vi "FitLorentzien.vi"() -> ()   [LabVIEW 2019]
uses:
  <vilib>/gmath/NumericalOptimization/Nonlinear Curve Fit LM formula string.vi
  <vilib>/Analysis/NI_AALBase.lvlib
  <vilib>/gmath/NI_Gmath.lvlib
panel:
  out "Residuals2":dbl
  out "NLCoeff2":dbl[](array[numeric])
  out "XY Graph 2":cluster{dbl[], "best nonlinear fit":dbl[]}[](graph)
  in  "Stop":bool
  out "Slide":u8(slide) scale=0.0..100.0
  out "Histogram Graph":T1(graph)
  in  "c":dbl
  out "XY Graph":cluster{dbl[], "Array":dbl[]}[](graph)
  out "NLCoeff":dbl[](array[numeric])
  out "Residuals":dbl[](array[numeric])
  out "Best Fit":dbl[](array[numeric])
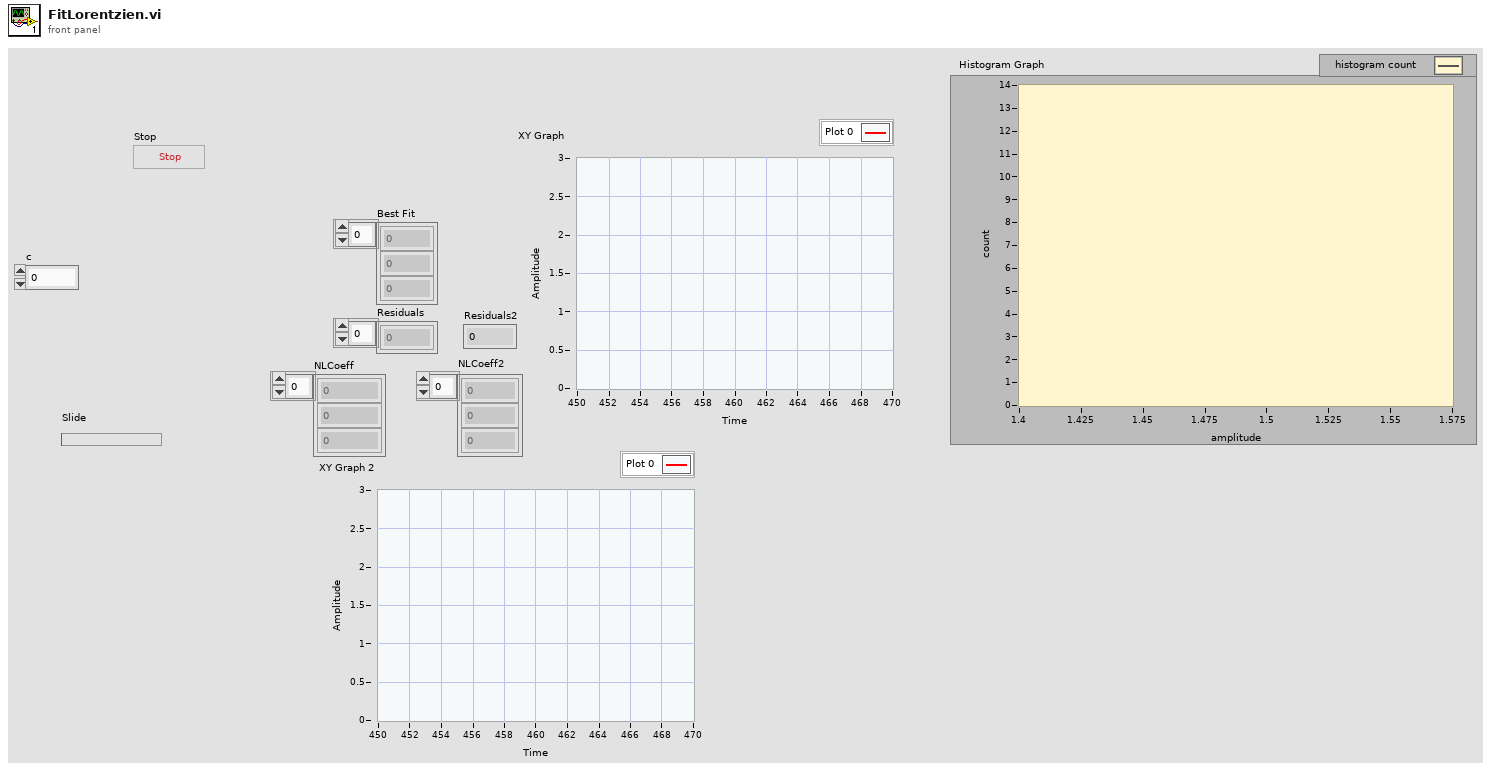
[diagram p1: front panel]
types:
  T1 = cluster{"X Values":dbl[], "Histogram: h(x)":i32[]}
  T2 = cluster{"model":string, "Parameters":string[], "x":string}
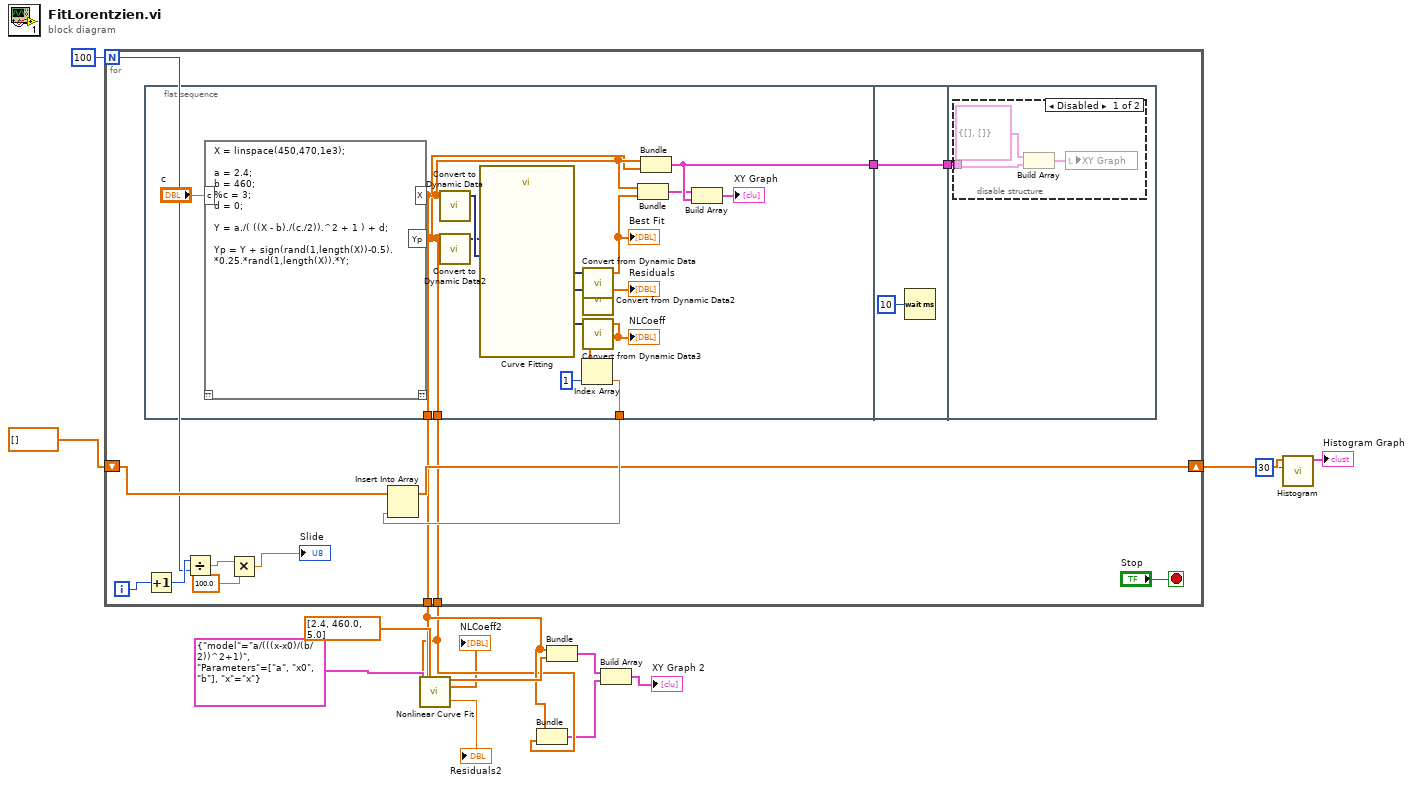
[diagram p0: block diagram]
diagram:
  n1 = for {
    N: 100 -> [w24]
    shift-right: [w27] -> w14
    shift-left: dbl[] [] -> [w29]
    tunnel: [w17] -> w6
    tunnel: [w16] -> w5
    i -> [w26]
    stop <- "Stop" stop-if-true
    n2 = flat-sequence {
      tunnel: [w45] -> w19
      tunnel: [w32] -> w28
      tunnel: [w31] -> w17
      tunnel: [w30] -> w16
      tunnel: w19 -> [w47]
      tunnel: [w47] -> w18
      tunnel: w18 -> [w48]
      frame #0 {
        n3 = script code="X = linspace(450,470,1e3);\n\na = 2.4;\nb = 460;\n%c = 3;\nd = 0;\n\nY = a./( ((X - b)./(c./2)).^2 + 1 ) + d;\n\nYp = Y + sign(rand(1,length(X))-0.5).*0.25.*rand(1,length(X)).*Y;"("c"="c") -> ("Yp"=w30:dbl[], "X"=w31:dbl[])  [unwired: 1 in, 1 out]
        n4 = call "Convert to Dynamic Data"("Array"=w31) -> ("Dynamic Data Type"=w44:dynamicdata)  [unwired: 3 in]
        n5 = call "Convert to Dynamic Data2"("Array"=w30) -> ("Dynamic Data Type"=w43:dynamicdata)  [unwired: 3 in]
        n6 = call "Curve Fitting"("Locations"=w44, "Signals"=w43) -> ("residual"=w41:dynamicdata, "best fit"=w42:dynamicdata, "non-linear coefficients"=w39:dynamicdata)  [unwired: 5 in, 2 out]
        n7 = call "Convert from Dynamic Data"("Dynamic Data Type"=w42) -> ("Array"=w38:dbl[])  [unwired: 3 in]
        "Best Fit" <- w38
        n8 = call "Convert from Dynamic Data2"("Dynamic Data Type"=w41) -> ("Array"=→"Residuals":dbl[])  [unwired: 3 in]
        n9 = call "Convert from Dynamic Data3"("Dynamic Data Type"=w39) -> ("Array"=w34:dbl[])  [unwired: 3 in]
        "NLCoeff" <- w34
        n10 = Index Array(array=w34, index=1) -> (element=w32:dbl)
        n11 = Bundle(w31, "Array"=w38) -> (w35:cluster{dbl[], "Array":dbl[]})  [unwired: 1 in]
        n12 = Bundle(w31, w30) -> (w45:cluster{dbl[], dbl[]})  [unwired: 1 in]
        n13 = Build Array(w35, w45) -> (→"XY Graph":cluster{dbl[], "Array":dbl[]}[])
      }
      frame #1 {
        n14 = Wait (ms)(milliseconds to wait=u32 10) -> ()  [unwired: 1 out]
      }
      frame #2 {
        n15 = disable-structure shown="Disabled" {
          disable-tunnel: w48 -> [w50 _]
          frame Disabled {
            n16 = Build Array(cluster{dbl[], dbl[]} {[], []} ("element"), w50) -> (w51:cluster{dbl[], dbl[]}[])
            n17 = local write "XY Graph"(w51) -> ()
          }
          frame Enabled {
          }
        }
      }
    }
    n18 = Increment(x=w26) -> (x+1=w25:i32)
    n19 = Divide(x=w25, y=w24) -> (x/y=w22:dbl)
    n20 = Multiply(x=w22, y=100.0) -> (x*y=→"Slide":dbl)
    n21 = Insert Into Array(array=w29, new element=w28) -> (w27:dbl[])  [unwired: 1 in]
  }
  n22 = call-poly <vilib>:"Nonlinear Curve Fit.vi"("Y"=w5, "initial parameters"=dbl[] [2.4, 460.0, 5.0], "X"=w6, "model description"=T2 {"model"="a/(((x-x0)/(b/2))^2+1)", "Parameters"=["a", "x0", "b"], "x"="x"}) -> ("best nonlinear fit"=w8:dbl[], "best fit parameters"=→"NLCoeff2":dbl[], "residue"=→"Residuals2":dbl)  [unwired: 7 in, 2 out]
  n23 = Bundle(w6, w5) -> (w4:cluster{dbl[], dbl[]})  [unwired: 1 in]
  n24 = Bundle(w6, "best nonlinear fit"=w8) -> (w7:cluster{dbl[], "best nonlinear fit":dbl[]})  [unwired: 1 in]
  n25 = Build Array(w7, w4) -> (→"XY Graph 2":cluster{dbl[], "best nonlinear fit":dbl[]}[])
  n26 = call <vilib>:"Histogram.vi"("intervals"=30, "X"=w14) -> ("Histogram Graph"=→"Histogram Graph":T1)  [unwired: 6 in, 3 out]
